vi "UI 1 Data Handler.vi"(8 "error in (no error)":errorcluster, 10 "UI 1 Data":T1, 11 "Current Val Data Set":cluster{"Acq Data":T5, "Post-Analysis Data":T6}) -> (0 "error out":errorcluster)   [LabVIEW 2014]
uses:
  Top Level/Shared Controls/UI Ref Arrays.ctl
  Top Level/Shared Controls/Acq Data.ctl
  Top Level/Shared Controls/Post-Analysis Data.ctl
  Private Controls/UI 1 Data.ctl
  Testing UI 1.lvlib
  Controller (Host)/Public Controls/Testing Select.ctl
  Controller (Host)/Controller (Host).lvlib
  Top Level/Shared Controls/Calculated Data.ctl
  File IO/Public Controls/General APU Info.ctl
  File IO/File IO.lvlib
  Top Level/Shared Controls/APU Setup File.ctl
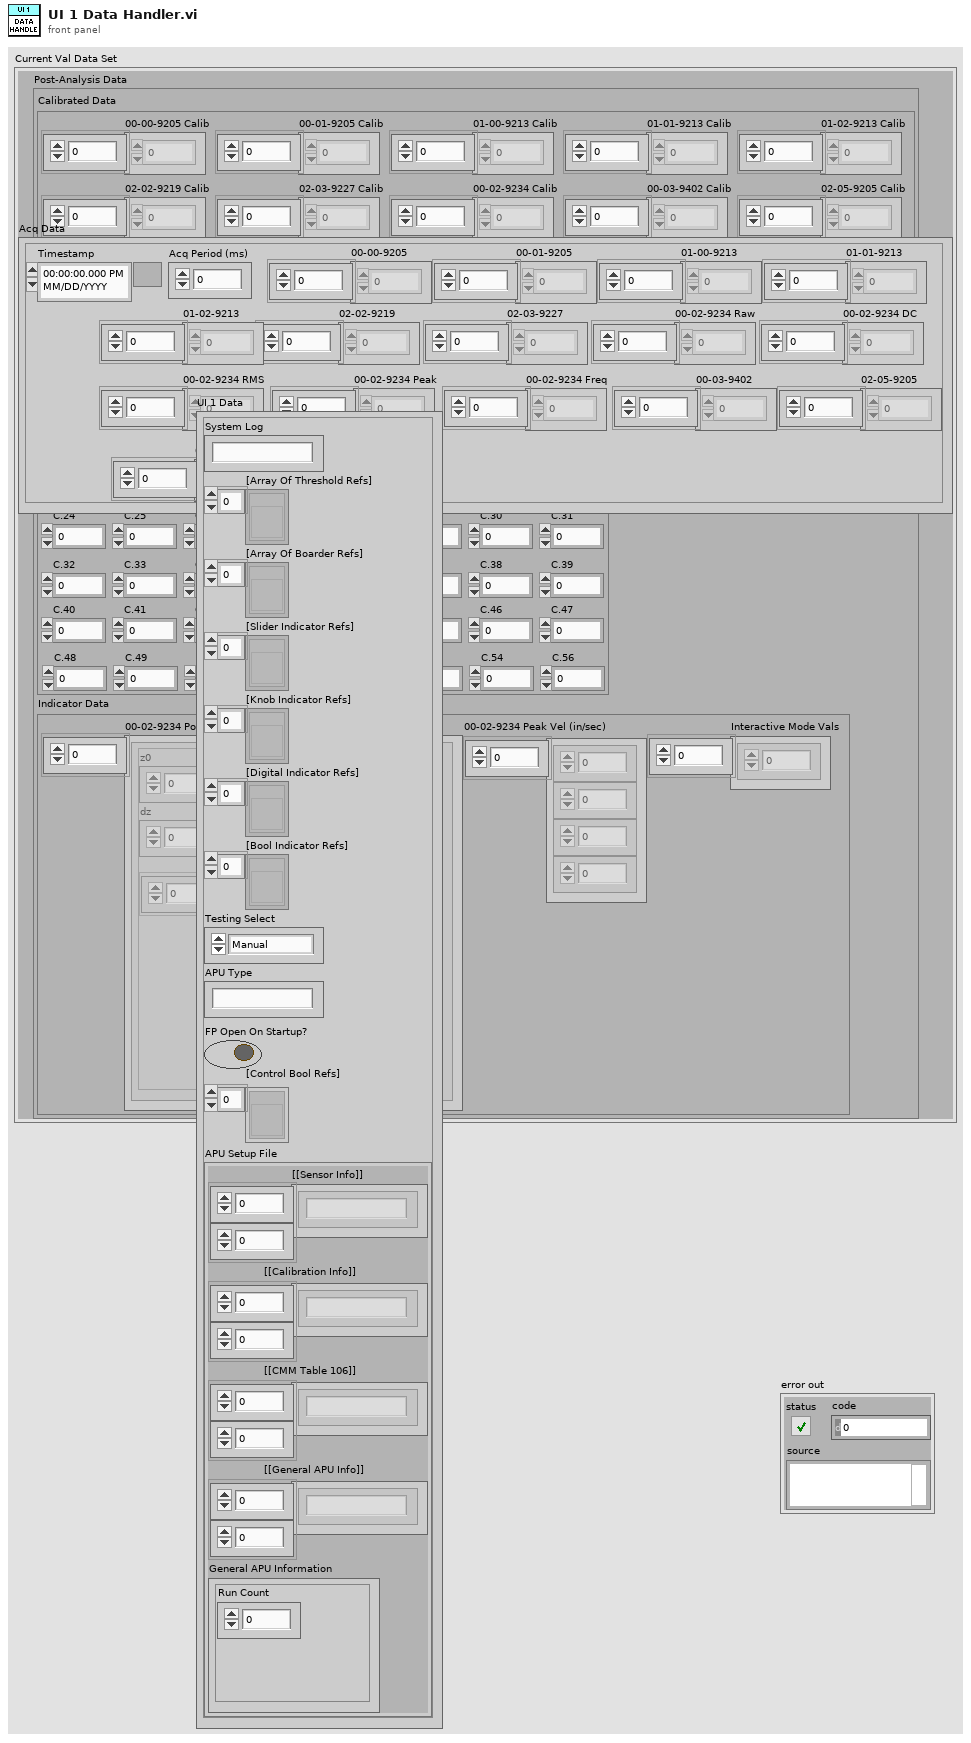
[diagram p1: front panel]
types:
  T1 = typedef "Testing UI 1.lvlib/UI 1 Data.ctl" = cluster{"System Log":string, "[Array Of Threshold Refs]":refnum<vi>[], "[Array Of Boarder Refs]":refnum<vi>[], "[Slider Indicator Refs]":refnum<vi>[], "[Knob Indicator Refs]":refnum<vi>[], "[Digital Indicator Refs]":refnum<vi>[], "[Bool Indicator Refs]":refnum<vi>[], "Testing Select":T2, "APU Type":string, "FP Open On Startup?":bool, "[Control Bool Refs]":refnum<vi>[], "APU Setup File":T3}
  T2 = typedef "Controller (Host).lvlib/Testing Select.ctl" = enum16{"Manual", "Interactive", "Automatic"}
  T3 = typedef "APU Setup File.ctl" = cluster{"[[Sensor Info]]":string[][], "[[Calibration Info]]":string[][], "[[CMM Table 106]]":string[][], "[[General APU Info]]":string[][], "General APU Information":T4}
  T4 = typedef "File IO.lvlib/General APU Info.ctl" = cluster{"Run Count":u64}
  T5 = typedef "Acq Data.ctl" = cluster{"Timestamp":timestamp, "Acq Period (ms)":i64, "00-00-9205":dbl[], "00-01-9205":dbl[], "01-00-9213":dbl[], "01-01-9213":dbl[], "01-02-9213":dbl[], "02-02-9219":dbl[], "02-03-9227":dbl[], "00-02-9234 Raw":dbl[], "00-02-9234 DC":dbl[], "00-02-9234 RMS":dbl[], "00-02-9234 Peak":dbl[], "00-02-9234 Freq":dbl[], "00-03-9402":dbl[], "02-05-9205":dbl[], "02-04-9871":dbl[]}
  T6 = typedef "Post-Analysis Data.ctl" = cluster{"Calibrated Data":cluster{"00-00-9205 Calib":dbl[], "00-01-9205 Calib":dbl[], "01-00-9213 Calib":dbl[], "01-01-9213 Calib":dbl[], "01-02-9213 Calib":dbl[], "02-02-9219 Calib":dbl[], "02-03-9227 Calib":dbl[], "00-02-9234 Calib":dbl[], "00-03-9402 Calib":dbl[], "02-05-9205 Calib":dbl[], "02-04-9871 2DArray":dbl[][]}, "Calculated Data":T7, "Indicator Data":cluster{"00-02-9234 Power Spectras":cluster{"z0":dbl, "dz":dbl, "waveforms":cluster{"f0":dbl, "df":dbl, "magnitude":dbl[]}[]}[], "00-02-9234 Peak Vel (in/sec)":dbl[], "Interactive Mode Vals":dbl[]}}
  T7 = typedef "Calculated Data.ctl" = cluster{"C.00":dbl, "C.01":dbl, "C.02":dbl, "C.03":dbl, "C.04":dbl, "C.05":dbl, "C.06":dbl, "C.07":dbl, "C.08":dbl, "C.09":dbl, "C.10":dbl, "C.11":dbl, "C.12":dbl, "C.13":dbl, "C.14":dbl, "C.15":dbl, "C.16":dbl, "C.17":dbl, "C.18":dbl, "C.19":dbl, "C.20":dbl, "C.21":dbl, "C.22":dbl, "C.23":dbl, "C.24":dbl, "C.25":dbl, "C.26":dbl, "C.27":dbl, "C.28":dbl, "C.29":dbl, "C.30":dbl, "C.31":dbl, "C.32":dbl, "C.33":dbl, "C.34":dbl, "C.35":dbl, "C.36":dbl, "C.37":dbl, "C.38":dbl, "C.39":dbl, "C.40":dbl, "C.41":dbl, "C.42":dbl, "C.43":dbl, "C.44":dbl, "C.45":dbl, "C.46":dbl, "C.47":dbl, "C.48":dbl, "C.49":dbl, "C.50":dbl, "C.51":dbl, "C.52":dbl, "C.53":dbl, "C.54":dbl, "C.56":dbl}
  T8 = typedef "UI Ref Arrays.ctl" = cluster{"[Slider Indicator Refs]":refnum<vi>[], "[Knob Indicator Refs]":refnum<vi>[], "[Digital Indicator Refs]":refnum<vi>[], "[[Sensor Info]]":string[][], "[Bool Indicator Refs]":refnum<vi>[]}
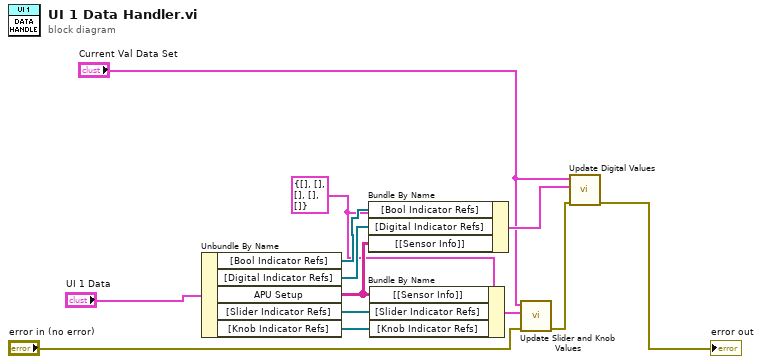
[diagram p0: block diagram]
diagram:
  w7 = T8 {"[Slider Indicator Refs]"=[], "[Knob Indicator Refs]"=[], "[Digital Indicator Refs]"=[], "[[Sensor Info]]"=[], "[Bool Indicator Refs]"=[]} ("Ref Data Array")
  n1 = Unbundle By Name("UI 1 Data") -> ("[Bool Indicator Refs]"=w13:refnum<vi>[], "[Digital Indicator Refs]"=w11:refnum<vi>[], "APU Setup"=w12:string[][], "[Slider Indicator Refs]"=w2:refnum<vi>[], "[Knob Indicator Refs]"=w3:refnum<vi>[])
  n2 = Bundle By Name(cluster=w7, "[Bool Indicator Refs]"=w13, "[Digital Indicator Refs]"=w11, "[[Sensor Info]]"=w12) -> (w10:T8)
  n3 = Bundle By Name(cluster=w7, "[[Sensor Info]]"=w12, "[Slider Indicator Refs]"=w2, "[Knob Indicator Refs]"=w3) -> (w8:T8)
  n4 = call "Update Slider and Knob Values.vi"("error in"="error in (no error)", "Ref Data Array"=w8, "Current Val Data Set"="Current Val Data Set") -> ("error out"=w5:errorcluster)  [unwired: 6 in, 2 out]
  n5 = call "Update Digital Values.vi"("error in (no error)"=w5, "Ref Data Array"=w10, "Current Val Data Set"="Current Val Data Set") -> ("error out"=→"error out":errorcluster)  [unwired: 6 in, 2 out]
